vi "MotionMagicExpoDutyCycle SetControl.vi"(0 "DeviceReference":T1, 1 "StopSendingOtherRequests":bool=TRUE, 2 "Position":dbl, 3 "EnableFOC":bool=TRUE, 4 "FeedForward":dbl, 5 "Slot":i32, 6 "OverrideBrakeDurNeutral":bool, 7 "error in":errorcluster, 8 "LimitForwardMotion":bool, 9 "LimitReverseMotion":bool, 18 "Update Frequency (Hz)":dbl=100.0) -> (20 "DeviceReference Out":T1, 27 "error out":errorcluster)   [LabVIEW 2023]
doc: "Requests Motion Magic® to target a final position using an exponential motion profile. Users can optionally provide a duty cycle feedforward.\nMotion Magic® Expo produces a motion profile in real-time while attempting to honor the Cruise Velocity (optional) and the mechanism kV and kA, specified via the Motion Magic® configuration values. Setting Cruise Velocity to 0 will allow the profile to run to the max possible velocity based on Expo_kV. This control mode does not use the Acceleration or Jerk configs. Target position can be changed on-the-fly and Motion Magic® will do its best to adjust the profile. This control mode is duty cycle based, so relevant closed-loop gains will use fractional duty cycle for the numerator: +1.0 represents full forward output."
uses:
  Users/Cory/Documents/PhoenixPro-LabVIEW-Generation/controls/DeviceReference.ctl
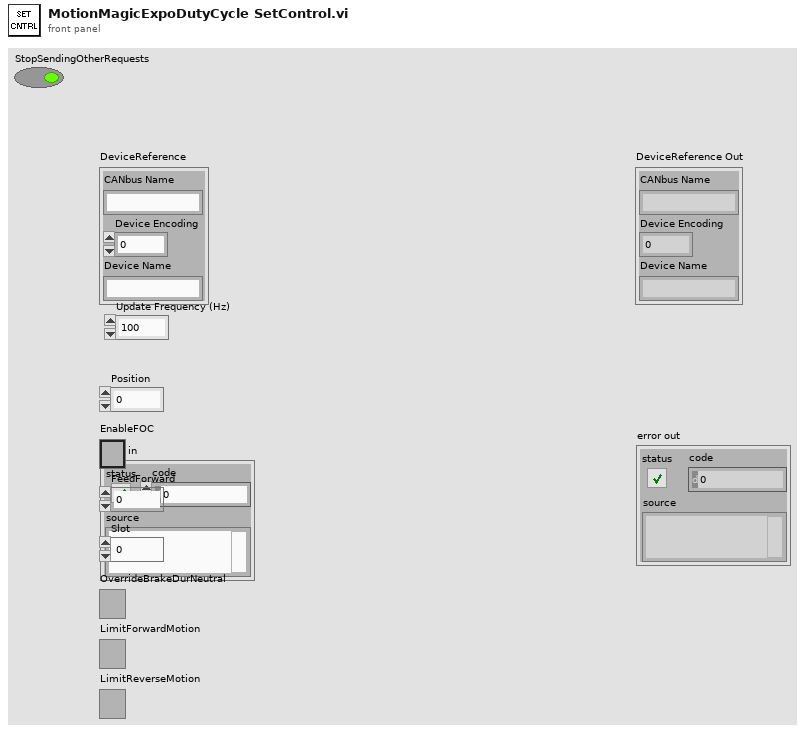
[diagram p1: front panel]
types:
  T1 = typedef "DeviceReference.ctl" = cluster{"CANbus Name":string, "Device Encoding":u32, "Device Name":string}
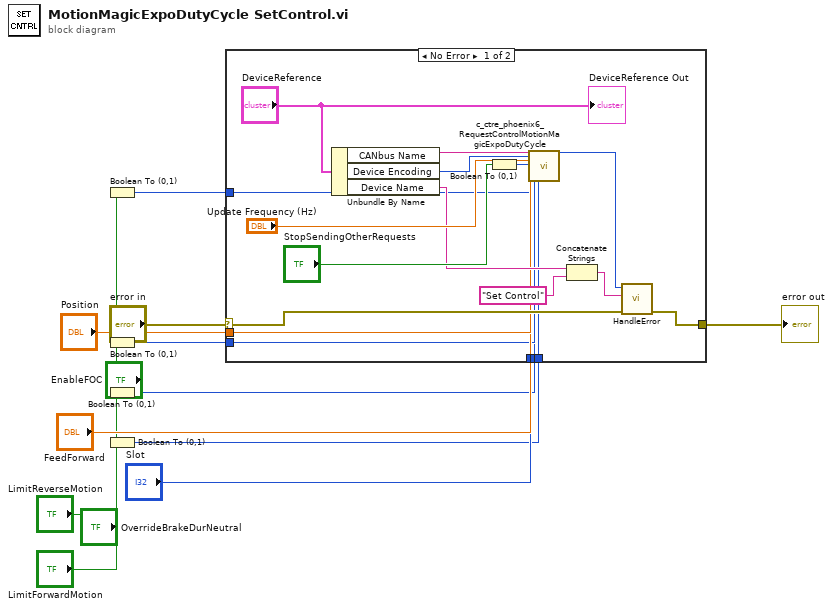
[diagram p0: block diagram]
diagram:
  n1 = Boolean To (0,1)(Boolean="EnableFOC") -> (0, 1=w9:i16)
  n2 = Boolean To (0,1)(Boolean="OverrideBrakeDurNeutral") -> (0, 1=w5:i16)
  n3 = Boolean To (0,1)(Boolean="LimitForwardMotion") -> (0, 1=w3:i16)
  n4 = Boolean To (0,1)(Boolean="LimitReverseMotion") -> (0, 1=w1:i16)
  n5 = case shown="No Error" "error in" {
    selector: "error in" -> [w25 w33]
    tunnel: [w24 w33] -> w12
    tunnel: "Position" -> [w20 _]
    tunnel: w9 -> [w19 _]
    tunnel: "FeedForward" -> [w18 _]
    tunnel: "Slot" -> [w17 _]
    tunnel: w5 -> [w16 _]
    tunnel: w3 -> [w15 _]
    tunnel: w1 -> [w14 _]
    frame No Error {
      n6 = Unbundle By Name("DeviceReference") -> ("CANbus Name"=w31:string, "Device Encoding"=w30:u32, "Device Name"=w23:string)
      n7 = Boolean To (0,1)(Boolean="StopSendingOtherRequests") -> (0, 1=w27:i16)
      n8 = call <vilib>:"c_ctre_phoenix6_RequestControlMotionMagicExpoDutyCycle.vi"("String 2"=w31, "Numeric 2"=w30, "Numeric 3"="Update Frequency (Hz)", "Numeric 4"=w27, "Numeric 5"=w20, "Numeric 6"=w19, "Numeric 7"=w18, "Numeric 8"=w17, "Numeric 9"=w16, "Numeric 10"=w15, "Numeric 11"=w14) -> ("Numeric"=w26:i32)  [unwired: 15 in, 1 out]
      n9 = Concatenate Strings(w23, "Set Control" ("origin")) -> (w21:string)
      n10 = call "HandleError.vi"("error in"=w25, "origin"=w21, "Status"=w26) -> ("error out"=w24:errorcluster)  [unwired: 8 in]
      "DeviceReference Out" <- "DeviceReference"
    }
    frame Error {
    }
  }
  "error out" <- w12
